vi "IsValidBaudrate.vi"(11 "Baud Rate":i32) -> (3 "x >= 0?":bool)   [LabVIEW 2026]
panel:
  in  "Valid Baudrates":i32[](array[numeric])=[10000, 20000, 50000, 100000, 125000, 250000, 500000, 800000, 1000000]
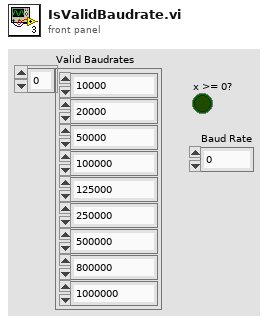
[diagram p1: front panel]
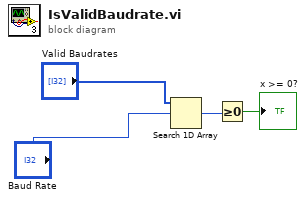
[diagram p0: block diagram]
diagram:
  n1 = Search 1D Array(1D array="Valid Baudrates", element="Baud Rate") -> (index of element=w2:i32)  [unwired: 1 in]
  n2 = Greater Or Equal To 0?(x=w2) -> (x >= 0?=→"x >= 0?":bool)
